vi "Entry Console View.vi"(8 "error in (no error)":errorcluster, 11 "View Model":T2) -> (0 "error out":errorcluster)   [LabVIEW 2017]
doc: "The interface via which user selects the car wash options to be executed by the Car Wash Controller.\n[Covers: UI2]"
uses:
  Model/Controls/View Model.ctl
  Model/Controls/Shared Model.ctl
  Error Handler/Controls/Error Model.ctl
  Error Handler/Controls/Error Message.ctl
  Error Handler/Controls/Error Type.ctl
  Configuration/Controls/Config Model.ctl
  Configuration/Controls/Config DB Message.ctl
  Configuration/Controls/Config DB Command.ctl
  Configuration/Controls/Config DB Overhead.ctl
  Configuration/Controls/Config DB Record1.ctl
  Controller/Controls/Controller Model.ctl
  Vehicle Position Simulation View/Controls/Vehicle - Position.ctl
  Controller/Controls/Controller Overhead.ctl
  Controller/Controls/Controller Wash Step.ctl
  Controller/Controls/Controller State.ctl
  Controls/Entry Console - Wash Step Select.ctl
  Controls/Entry Console - GUI References.ctl
panel:
  in  "Wash Step Select":T1
  in  "Start":bool
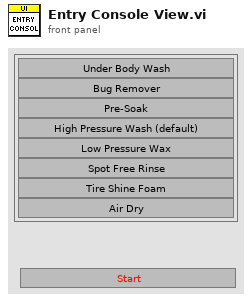
[diagram p1: front panel]
types:
  T1 = typedef "Entry Console - Wash Step Select.ctl" = cluster{"Under Body Wash":bool, "Bug Remover":bool, "Pre-Soak":bool, "High Pressure Wash":bool, "Low Pressure Wax":bool, "Spot Free Rinse":bool, "Tire Shine Foam":bool, "Air Dry":bool}
  T2 = typedef "View Model.ctl" = cluster{"Shared Model":T3, "Error Model":T4, "Config Model":T5, "Controller Model":T6}
  T3 = typedef "Shared Model.ctl" = cluster{"Stop":refnum<user-event>, "Stop DVR":refnum<data-value>}
  T4 = typedef "Error Model.ctl" = cluster{"Error":refnum<user-event>}
  T5 = typedef "Config Model.ctl" = cluster{"Config":refnum<user-event>, "Config DVR":refnum<data-value>}
  T6 = typedef "Controller Model.ctl" = cluster{"Position Change":refnum<user-event>, "Overhead DVR":refnum<data-value>, "Wash Cycle Start":refnum<user-event>, "Wash Step Start":refnum<user-event>, "Out Of Position":refnum<user-event>, "Views Command":refnum<user-event>}
  T7 = typedef "Entry Console - GUI References.ctl" = cluster{"Start":refnum<vi>, "Wash Step Select":refnum<vi>}
  T8 = enum8{"Enabled", "Disabled", "Disabled and Grayed Out"}
  T9 = typedef "Error Type.ctl" = enum16{"Minor Error", "Wash Cycle Error", "System Error", "Unknown"}
  T10 = typedef "Controller State.ctl" = enum16{"Initial", "Wait for Start", "Wash Cycle Start", "Wash Cycle Complete", "Wash Step Start", "Wash Step Execute", "Wash Step Complete", "Wait for Vehicle Position", "Wash Exit", "Wash Abort/Terminate"}
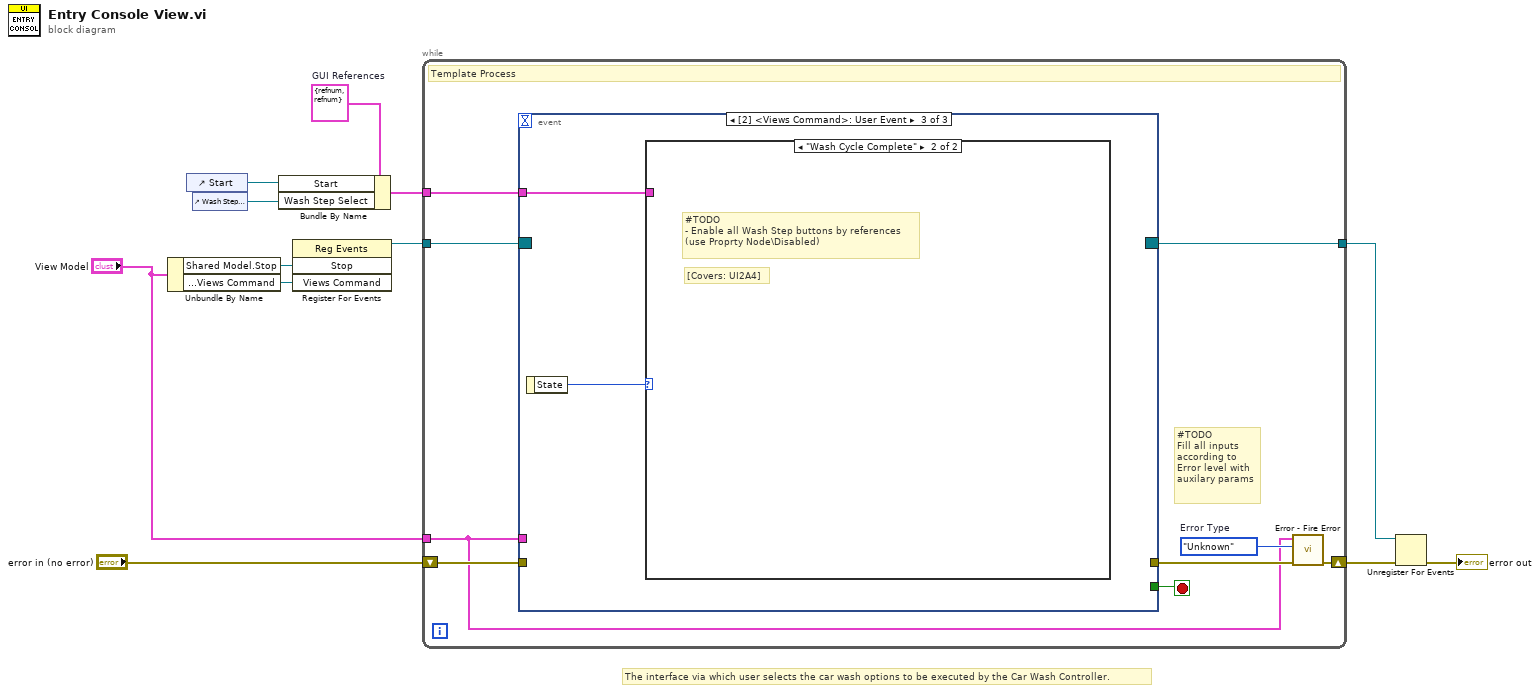
[diagram p0: block diagram]
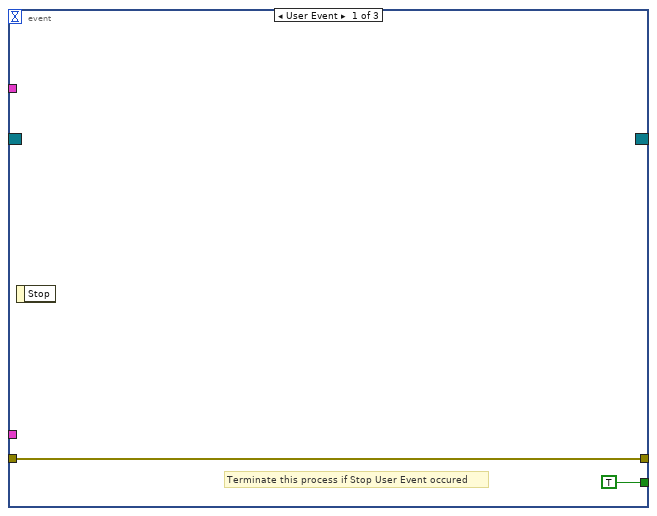
[diagram p2: hidden frame]
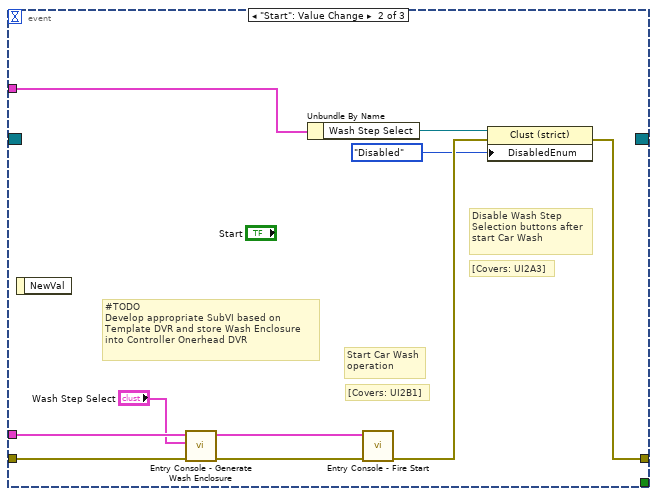
[diagram p3: hidden frame]
diagram:
  w5 = T7 {"Start"=refnum, "Wash Step Select"=refnum}  # GUI References
  # "The interface via which user selects the car wash options to be executed by the Car Wash Controller."
  n1 = Unbundle By Name("View Model") -> ("Shared Model.Stop"=w12:refnum<user-event>, "Controller Model.Views Command"=w1:refnum<user-event>)
  n2 = control-ref of="Start"() -> (w4:refnum<vi>)
  n3 = control-ref of="Wash Step Select"() -> (w3:refnum<vi>)
  n4 = Bundle By Name(cluster=w5, "Start"=w4, "Wash Step Select"=w3) -> (w2:T7)
  n5 = register-events(w12, w1) -> (reference out=w11:refnum<event-registration>)  [unwired: 2 in, 1 out]
  n6 = while {
    tunnel: w11 -> [w21]
    shift-right: [w16] -> w9
    shift-left: "error in (no error)" -> [w20]
    tunnel: [w19] -> w7
    tunnel: "View Model" -> [w14]
    tunnel: w2 -> [w13]
    stop <- w18 stop-if-true
    w15 = Error_Type."Unknown"  # Error Type
    # "#TODO\nFill all inputs\naccording to \nError level with\nauxilary params"
    # "Template Process"
    n7 = event shown="[2] <Views Command>: User Event" {
      selector: w21 -> [_ _ _]
      dyn-events: [_ _ _] -> w19
      timeout: _ -> [_ _ _]
      tunnel: w20 -> [w23 w33 _]
      tunnel: [w23 w25 _] -> w17
      tunnel: w14 -> [_ w32 _]
      tunnel: [TRUE _ _] -> w18
      tunnel: w13 -> [_ w28 w34]
      event User Event {
        # "Terminate this process if Stop User Event occured"
        n8 = event-data() -> ()  [unwired: 1 in, 1 out]
      }
      event "Start": Value Change {
        # "[Covers: UI2B1]"
        # "Start Car Wash\noperation"
        # "[Covers: UI2A3]"
        # "Disable Wash Step \nSelection buttons after\nstart Car Wash"
        # "#TODO\nDevelop appropriate SubVI based on\nTemplate DVR and store Wash Enclosure\ninto Controller Onerhead DVR"
        n9 = event-data() -> ()  [unwired: 1 in, 1 out]
        n10 = call "Entry Console - Generate Wash Enclosure.vi"("error in (no error)"=w33, "Wash Step Selection buttons"="Wash Step Select", "View Model"=w32) -> ("error out"=w30:errorcluster, "View Model"=w29:T2)  [unwired: 6 in, 1 out]
        n11 = Unbundle By Name(w28) -> ("Wash Step Select"=w27:refnum<vi>)
        n12 = call "Entry Console - Fire Start.vi"("error in (no error)"=w30, "View Model"=w29) -> ("error out"=w26:errorcluster)  [unwired: 8 in, 1 out]
        n13 = property class="Clust (strict)"(reference=w27, error in=w26, "DisabledEnum"=T8."Disabled" ("Disabled")) -> (error out=w25:errorcluster)  [unwired: 1 out]
      }
      event User Event {
        n14 = event-data() -> ("State"=w35:T10)  [unwired: 1 in]
        n15 = case shown="\"Wash Cycle Complete\"" w35 {
          tunnel: w34 -> [_ _]
          frame Default {
          }
          frame "Wash Cycle Complete" {
            # "[Covers: UI2A4]"
            # "#TODO\n- Enable all Wash Step buttons by references\n(use Proprty Node\\Disabled)"
          }
        }
      }
    }
    n16 = call "Error - Fire Error.vi"("error in (no error)"=w17, "Error Type"=w15, "View Model"=w14) -> ("error out"=w16:errorcluster)  [unwired: 7 in, 1 out]
  }
  n17 = Unregister For Events(event registration refnum=w7, error in=w9) -> (error out=→"error out":errorcluster)
